vi "Data Section Page GUID.vi"() -> (3 "Data GUID":string="bcfbab85-abaa-4292-95db-a76142f82350")   [LabVIEW 2020, in "DSF Shared.lvlib"]
uses:
  DSF Shared.lvlib
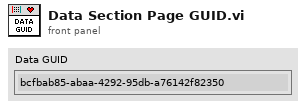
[diagram p1: front panel]
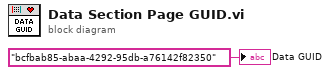
[diagram p0: block diagram]
diagram:
  "Data GUID" <- "bcfbab85-abaa-4292-95db-a76142f82350" ("Data Sharing Framework")
